vi "Temp_write.vi"() -> ()   [LabVIEW 2020]
panel:
  in  "data":waveform(dbl)[](array[waveform])
  in  "name or relative path":path
  in  "operation (0:open)":T1(ring)=enum."open or create"
  in  "group name in (Untitled)":string="Data"
  in  "channel name(s) in (Untitled)":string[](array[string])
  in  "stop":bool
  in  "file format version (2.0)":enum16{"1.0", "2.0"}(ring)
  in  "file path":path
  out "error out":errorcluster
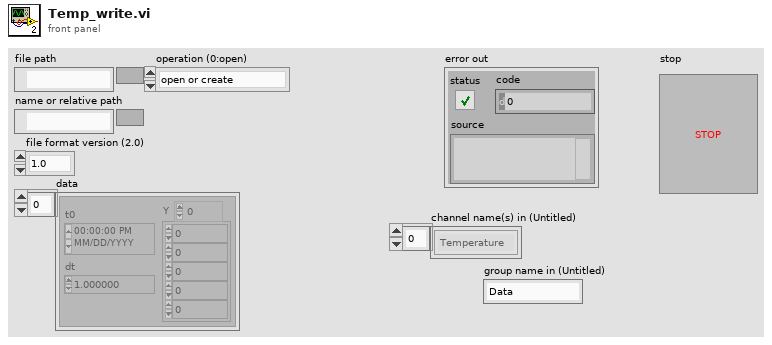
[diagram p1: front panel]
types:
  T1 = enum16{"open", "open or create", "create or replace", "create", "open (read-only)"}
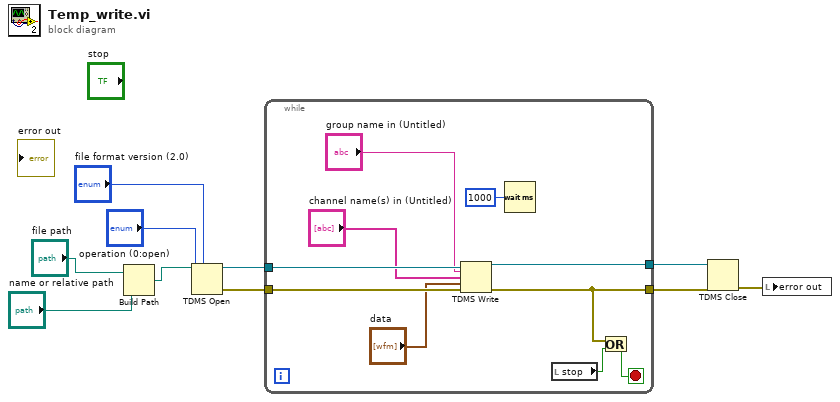
[diagram p0: block diagram]
diagram:
  n1 = Build Path(base path="file path", name or relative path="name or relative path") -> (appended path=w3:path)
  n2 = TDMS Open(7:"file format version (2.0)", 10:"operation (0:open)", 11:w3) -> (0:w8:errorcluster, 3:w6:refnum<k34>)  [unwired: 4 in]
  n3 = while {
    tunnel: [w13] -> w9
    tunnel: w8 -> [w19]
    tunnel: w6 -> [w18]
    tunnel: [w17] -> w5
    stop <- w12 stop-if-true
    n4 = TDMS Write(0:w18, 5:"group name in (Untitled)", 7:"channel name(s) in (Untitled)", 9:"data", 11:w19) -> (4:w17:refnum<k34>, 15:w13:errorcluster)  [unwired: 1 in, 2 out]
    n5 = Wait (ms)(milliseconds to wait=u32 1000) -> ()  [unwired: 1 out]
    n6 = local read "stop"() -> (w14:bool)
    n7 = Or(x=w13, y=w14) -> (x .or. y?=w12:bool)
  }
  n8 = TDMS Close(8:w9, 11:w5) -> (0:w10:errorcluster)  [unwired: 1 out]
  n9 = local write "error out"(w10) -> ()
